vi "Launcher.vi"() -> ()   [LabVIEW 2019]
uses:
  Launcher State.ctl
panel:
  out "Enum":T1
  out "Engines Firing":bool
  out "Engine Shutoff Timer":dbl
  out "Countdown":dbl
  in  "Abort":bool
  in  "Launch":bool
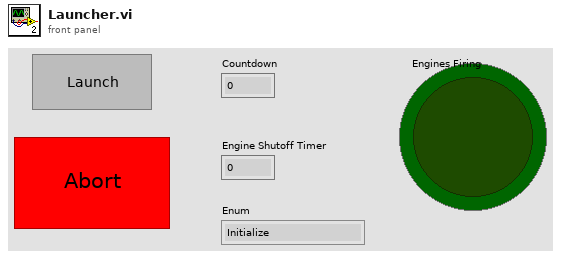
[diagram p1: front panel]
types:
  T1 = typedef "Launcher State.ctl" = enum16{"Initialize", "Ready", "Start Countdown", "Countdown", "Start Firing", "Firing", "Engine Stop", "Abort"}
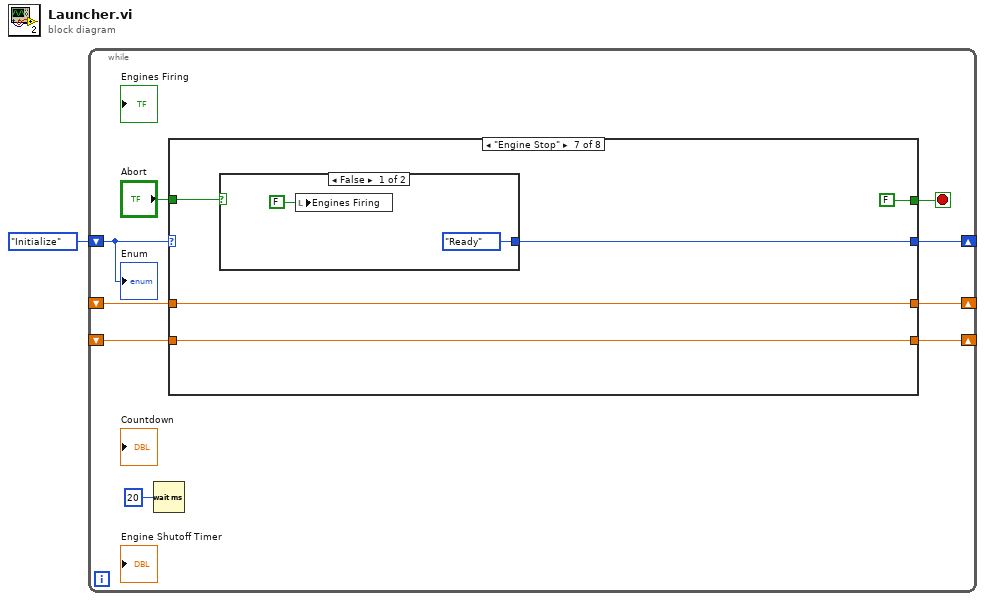
[diagram p0: block diagram]
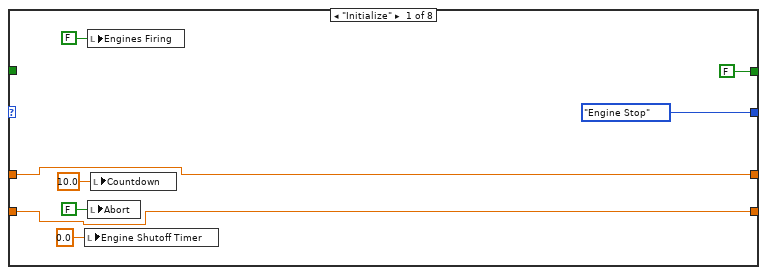
[diagram p2: hidden frame]
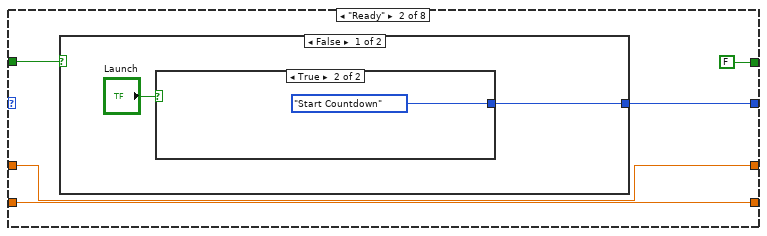
[diagram p3: hidden frame]
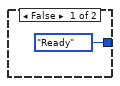
[diagram p4: hidden frame]
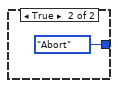
[diagram p5: hidden frame]
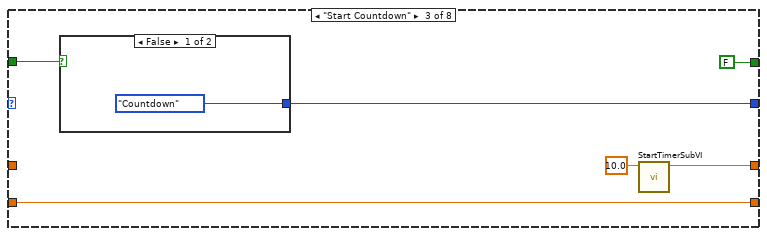
[diagram p6: hidden frame]
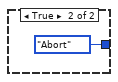
[diagram p7: hidden frame]
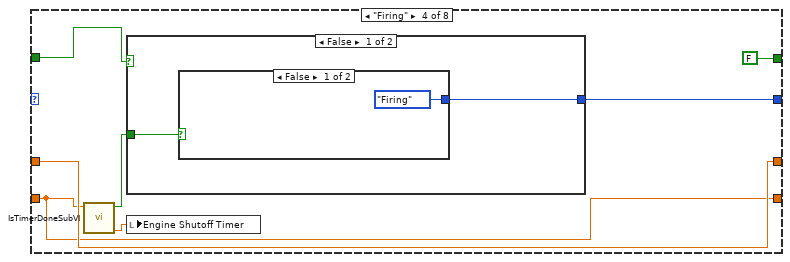
[diagram p8: hidden frame]
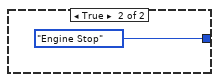
[diagram p9: hidden frame]
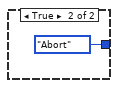
[diagram p10: hidden frame]
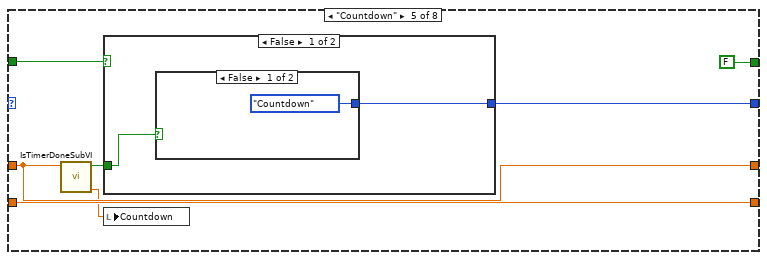
[diagram p11: hidden frame]
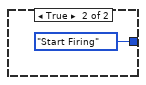
[diagram p12: hidden frame]
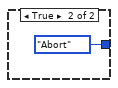
[diagram p13: hidden frame]
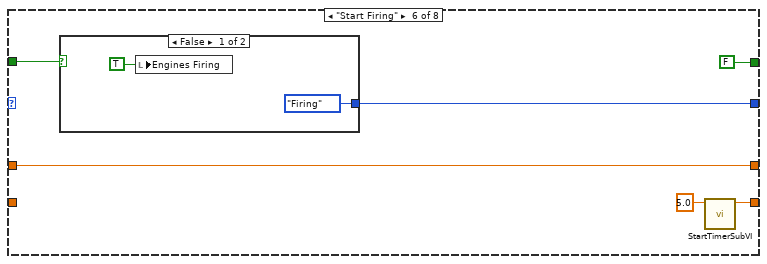
[diagram p14: hidden frame]
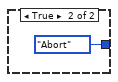
[diagram p15: hidden frame]
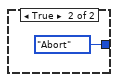
[diagram p16: hidden frame]
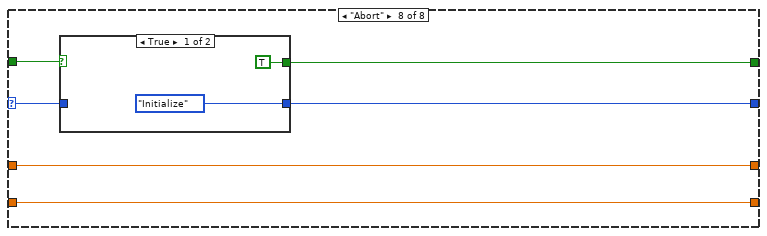
[diagram p17: hidden frame]
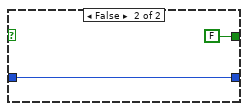
[diagram p18: hidden frame]
diagram:
  n1 = while {
    shift-right: [w8] -> _
    shift-left: Launcher_State."Initialize" ("Enum") -> [w9]
    shift-right: [w6] -> _
    shift-left: _ -> [w3]
    shift-right: [w5] -> _
    shift-left: _ -> [w4]
    stop <- w2 stop-if-true
    n2 = Wait (ms)(milliseconds to wait=u32 20) -> ()  [unwired: 1 out]
    n3 = case shown="\"Engine Stop\"" w9 {
      selector: w9 -> [_ _ _ _ _ _ _ w79]
      tunnel: [Launcher_State."Engine Stop" ("Enum") w22 w33 w39 w54 w65 w73 w82] -> w8
      tunnel: "Abort" -> [_ w23 w34 w43 w55 w66 w74 w83]
      tunnel: [w14 w21 w31 w42 w52 w64 w72 w81] -> w6
      tunnel: w3 -> [w14 w21 _ w42 w52 w64 w72 w81]
      tunnel: [w13 w20 w30 w41 w51 w62 w71 w80] -> w5
      tunnel: w4 -> [w13 w20 w30 w41 w51 _ w71 w80]
      tunnel: [FALSE FALSE FALSE FALSE FALSE FALSE FALSE w78] -> w2
      frame "Initialize" {
        n4 = local write "Engine Shutoff Timer"(0.0 ("Engine Shutoff Timer")) -> ()
        n5 = local write "Engines Firing"(FALSE ("Engines Firing")) -> ()
        n6 = local write "Abort"(FALSE ("Abort")) -> ()
        n7 = local write "Countdown"(10.0 ("Countdown")) -> ()
      }
      frame "Ready" {
        n8 = case shown="False" w23 {
          tunnel: [w24 Launcher_State."Abort" ("Enum")] -> w22
          frame False {
            n9 = case shown="True" "Launch" {
              tunnel: [Launcher_State."Ready" ("Enum") Launcher_State."Start Countdown" ("Enum")] -> w24
              frame False {
              }
              frame True {
              }
            }
          }
          frame True {
          }
        }
      }
      frame "Start Countdown" {
        n10 = case shown="False" w34 {
          tunnel: [Launcher_State."Countdown" ("Enum") Launcher_State."Abort" ("Enum")] -> w33
          frame False {
          }
          frame True {
          }
        }
        n11 = call "StartTimerSubVI.vi"("Wait Time (Seconds)"=10.0) -> ("End Time (Seconds)"=w31:dbl)  [unwired: 10 in]
      }
      frame "Firing" {
        n12 = call "IsTimerDoneSubVI.vi"("End Time (Seconds)"=w41) -> ("Time Done"=w40:bool, "Time Left"=w38:dbl)  [unwired: 7 in]
        n13 = case shown="False" w43 {
          tunnel: w40 -> [w45 _]
          tunnel: [w44 Launcher_State."Abort" ("Enum")] -> w39
          frame False {
            n14 = case shown="False" w45 {
              tunnel: [Launcher_State."Firing" ("Enum") Launcher_State."Engine Stop" ("Enum")] -> w44
              frame False {
              }
              frame True {
              }
            }
          }
          frame True {
          }
        }
        n15 = local write "Engine Shutoff Timer"(w38) -> ()
      }
      frame "Countdown" {
        n16 = call "IsTimerDoneSubVI.vi"("End Time (Seconds)"=w52) -> ("Time Done"=w53:bool, "Time Left"=w50:dbl)  [unwired: 7 in]
        n17 = case shown="False" w55 {
          tunnel: [w56 Launcher_State."Abort" ("Enum")] -> w54
          tunnel: w53 -> [w57 _]
          frame False {
            n18 = case shown="False" w57 {
              tunnel: [Launcher_State."Countdown" ("Enum") Launcher_State."Start Firing" ("Enum")] -> w56
              frame False {
              }
              frame True {
              }
            }
          }
          frame True {
          }
        }
        n19 = local write "Countdown"(w50) -> ()
      }
      frame "Start Firing" {
        n20 = case shown="False" w66 {
          tunnel: [Launcher_State."Firing" ("Enum") Launcher_State."Abort" ("Enum")] -> w65
          frame False {
            n21 = local write "Engines Firing"(TRUE ("Engines Firing")) -> ()
          }
          frame True {
          }
        }
        n22 = call "StartTimerSubVI.vi"("Wait Time (Seconds)"=5.0) -> ("End Time (Seconds)"=w62:dbl)  [unwired: 10 in]
      }
      frame "Engine Stop" {
        n23 = case shown="False" w74 {
          tunnel: [Launcher_State."Ready" ("Enum") Launcher_State."Abort" ("Enum")] -> w73
          frame False {
            n24 = local write "Engines Firing"(FALSE ("Engines Firing")) -> ()
          }
          frame True {
          }
        }
      }
      frame "Abort" {
        n25 = case shown="True" w83 {
          tunnel: [Launcher_State."Initialize" ("Enum") w87] -> w82
          tunnel: w79 -> [_ w87]
          tunnel: [TRUE FALSE] -> w78
          frame True {
          }
          frame False {
          }
        }
      }
    }
    "Enum" <- w9
  }
